vi "Create All Message Queues.vi"(8 "error in (no error)":errorcluster) -> (0 "error out":errorcluster, 3 "Message Queues out":T1)   [LabVIEW 2019, in "Message Queue.lvlib"]
doc: "This VI creates and initializes all the message queues for your application. If your application requires more than one message queue, right-click the \"Message Queues\" constant above and select Open Type Def. Add the new Message Queue(s) to the type definition, then initialize them in this VI."
uses:
  Message Queue.lvlib
  All Message Queues.ctl
  Message Cluster.ctl
  Enqueue Message (Single).vi
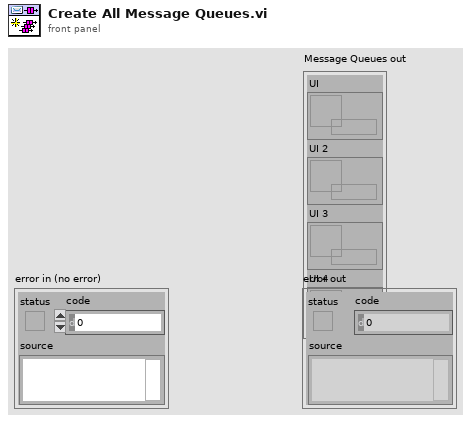
[diagram p1: front panel]
types:
  T1 = typedef "Message Queue.lvlib/All Message Queues.ctl" = cluster{"UI":refnum<queue>, "UI 2":refnum<queue>, "UI 3":refnum<queue>, "UI 4":refnum<queue>}
  T2 = cluster{"[0]":refnum<queue>, "[1]":refnum<queue>, "[2]":refnum<queue>, "[3]":refnum<queue>}
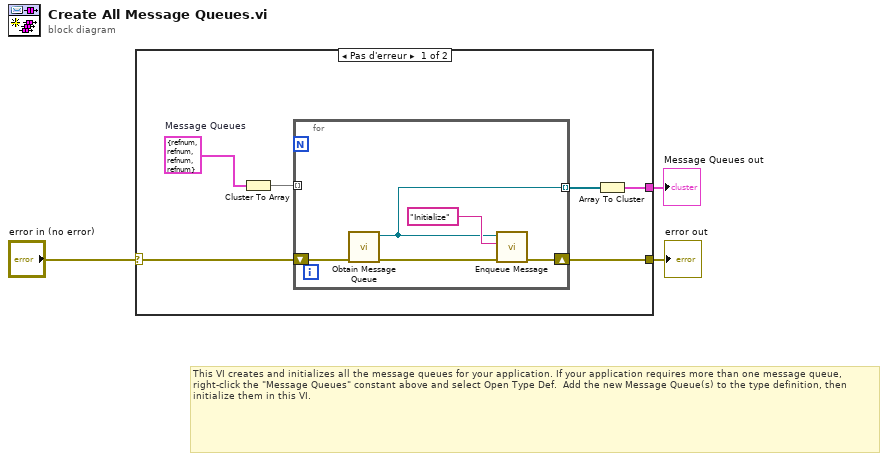
[diagram p0: block diagram]
diagram:
  # "This VI creates and initializes all the message queues for your application. If your application requires more than one message queue, right-click the \"Message Queues\" constant above and select Open Type Def.  Add the new Message Queue(s) to the type definition, then initialize them in this VI."
  n1 = case shown="Pas d'erreur" "error in (no error)" {
    selector: "error in (no error)" -> [w8 w15]
    tunnel: [w9 w15] -> w3
    tunnel: [w5 _] -> w1
    frame No Error {
      w7 = T1 {"UI"=refnum, "UI 2"=refnum, "UI 3"=refnum, "UI 4"=refnum}  # Message Queues
      n2 = Cluster To Array(cluster=w7) -> (array=w6:refnum<queue>[])
      n3 = for {
        shift-right: [w14] -> w9
        shift-left: w8 -> [w13]
        tunnel: w6 -> [_] mode=indexing
        tunnel: [w10] -> w4 mode=indexing
        n4 = call "Obtain Message Queue.vi"("error in (no error)"=w13) -> ("error out"=w12:errorcluster, "Message Queue"=w10:refnum<queue>)  [unwired: 9 in]
        n5 = call-poly "Enqueue Message.vi"("error in (no error)"=w12, "Message"="Initialize", "Message Queue"=w10) -> ("error out"=w14:errorcluster)  [unwired: 7 in, 1 out]
      }
      n6 = Array To Cluster(array=w4) -> (cluster=w5:T2)
    }
    frame Error {
    }
  }
  "Message Queues out" <- w1
  "error out" <- w3
